vi "Cliente_DSTP.vi"() -> ()   [LabVIEW 2016]
panel:
  in  "variant":variant
  out "Boolean":bool
  out "Waveform Chart":dbl(graph)
  in  "Stop Button":bool
  in  "Knob":dbl(knob) scale=0.0..10.0
  # "CLIENTE"
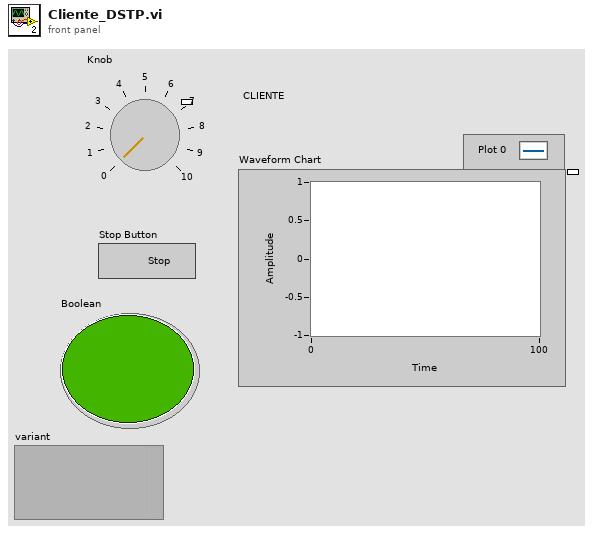
[diagram p1: front panel]
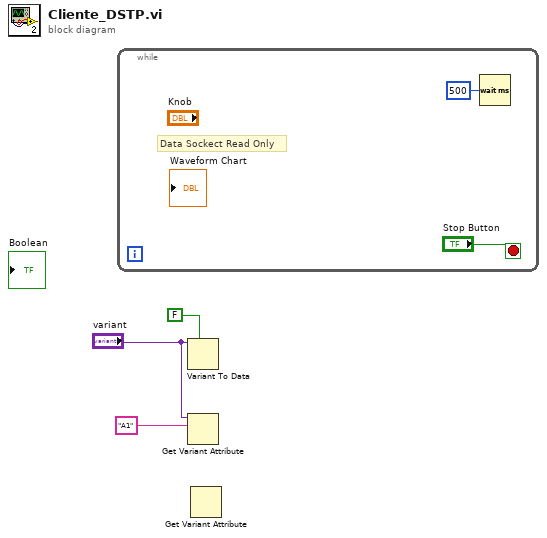
[diagram p0: block diagram]
diagram:
  n1 = while {
    stop <- "Stop Button" stop-if-true
    # "Data Sockect Read Only"
    n2 = Wait (ms)(milliseconds to wait=u32 500) -> ()  [unwired: 1 out]
  }
  n3 = Variant To Data(type=FALSE, Variant="variant") -> ()  [unwired: 1 in, 2 out]
  n4 = Get Variant Attribute(Variant="variant", name="A1") -> ()  [unwired: 2 in, 4 out]
  n5 = Get Variant Attribute() -> ()  [unwired: 4 in, 4 out]
